vi "Action Send Trigger.vi"(0 "VISA resource name":refnum<visa-resource-name>, 5 "error in (no error)":errorcluster) -> (14 "VISA resource name out":refnum<visa-resource-name>, 19 "error out":errorcluster)   [LabVIEW 2021, in "Keithley 2000.lvlib"]
doc: "This VI sends a manual (bus) trigger to the instrument."
uses:
  Keithley 2000.lvlib
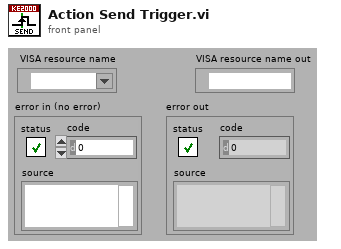
[diagram p1: front panel]
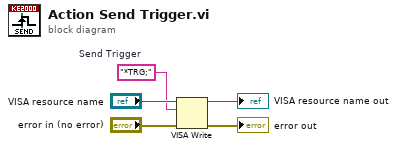
[diagram p0: block diagram]
diagram:
  w3 = "*TRG;"  # Send Trigger
  n1 = VISA Write(VISA resource name="VISA resource name", write buffer=w3, error in (no error)="error in (no error)") -> (VISA resource name out=→"VISA resource name out":refnum<visa-resource-name>, error out=→"error out":errorcluster)  [unwired: 1 out]
